vi "Lockin.DAQ.Read AI and Write AO.vi"(8 "error in (no error)":errorcluster, 11 "Lockin.DAQ in":refnum<class "Instrument.DAQ.lvclass">) -> (0 "error out":errorcluster, 3 "Lockin.DAQ out":refnum<class "Instrument.DAQ.lvclass">)   [LabVIEW 2019, in "Instrument.DAQ.lvclass"]
uses:
  Instrument.DAQ.lvclass
panel:
  out "AO":u32
  out "AI":u32
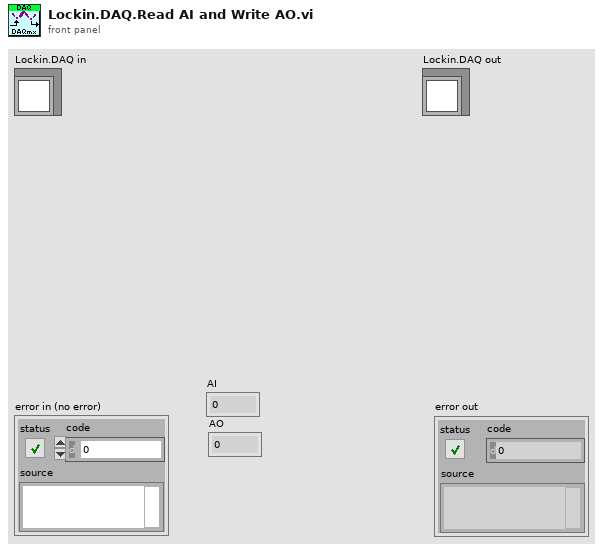
[diagram p1: front panel]
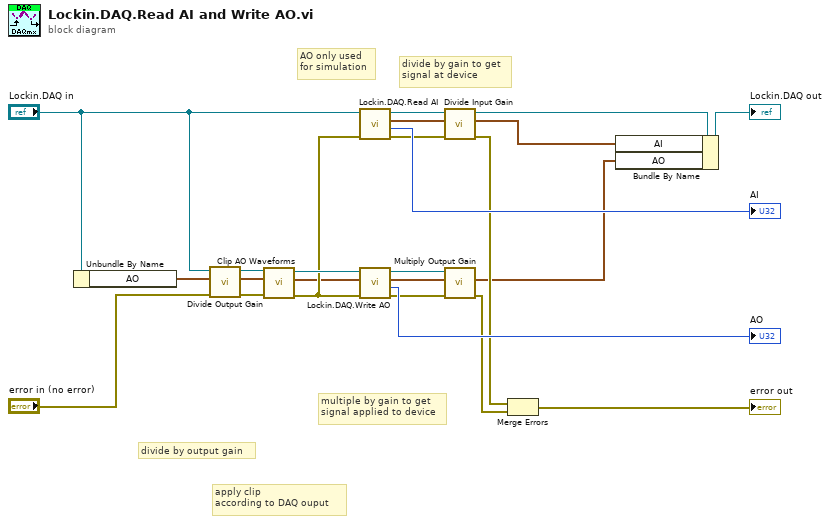
[diagram p0: block diagram]
diagram:
  # "divide by gain to get\nsignal at device"
  # "multiple by gain to get\nsignal applied to device"
  # "apply clip\naccording to DAQ ouput"
  # "divide by output gain"
  # "AO only used\nfor simulation"
  n1 = Unbundle By Name("Lockin.DAQ in") -> ("AO"=w5:waveform(dbl)[])
  n2 = call "Divide Output Gain.vi"("error in (no error)"="error in (no error)", "WFM in"=w5, "Lockin.DAQ"="Lockin.DAQ in") -> ("error out"=w20:errorcluster, "WFM out"=w22:waveform(dbl)[], "Lockin.DAQ out"=w21:refnum<class "Instrument.DAQ.lvclass">)  [unwired: 6 in]
  n3 = call "Clip AO Waveforms.vi"("error in (no error)"=w20, "AO []"=w22, "Lockin.DAQ in"=w21) -> ("error out"=w18:errorcluster, "Clipped AO []"=w7:waveform(dbl)[], "Lockin.DAQ out"=w19:refnum<class "Instrument.DAQ.lvclass">)  [unwired: 6 in]
  n4 = call "Lockin.DAQ.Read AI.vi"("error in (no error)"=w18, "Lockin.DAQ in"="Lockin.DAQ in") -> ("error out"=w14:errorcluster, "AI time (ms)"=→"AI":u32, "AI []"=w16:waveform(dbl)[], "Lockin.DAQ out"=w15:refnum<class "Instrument.DAQ.lvclass">)  [unwired: 6 in]
  n5 = call "Lockin.DAQ.Write AO.vi"("error in (no error)"=w18, "AO []"=w7, "Lockin.DAQ in"=w19) -> ("error out"=w13:errorcluster, "AO time (ms)"=→"AO":u32, "AO out []"=w11:waveform(dbl)[], "Lockin.DAQ out"=w17:refnum<class "Instrument.DAQ.lvclass">)  [unwired: 5 in]
  n6 = call "Divide Input Gain.vi"("error in (no error)"=w14, "WFM in"=w16, "Lockin.DAQ"=w15) -> ("error out"=w9:errorcluster, "WFM out"=w2:waveform(dbl)[], "Lockin.DAQ out"=w4:refnum<class "Instrument.DAQ.lvclass">)  [unwired: 6 in]
  n7 = call "Multiply Output Gain.vi"("error in (no error)"=w13, "WFM in"=w11, "Lockin.DAQ"=w17) -> ("error out"=w8:errorcluster, "WFM out"=w1:waveform(dbl)[])  [unwired: 6 in, 1 out]
  n8 = Merge Errors(w9, w8) -> (→"error out":errorcluster)
  n9 = Bundle By Name(cluster=w4, "AI"=w2, "AO"=w1) -> (→"Lockin.DAQ out":refnum<class "Instrument.DAQ.lvclass">)
